vi "Get Service Description.vi"(0 "Room Service Base in":refnum<class "Room Service Base.lvclass">, 11 "error in (no error)":errorcluster) -> (4 "Room Service Base out":refnum<class "Room Service Base.lvclass">, 6 "Service Description":string, 15 "error out":errorcluster)   [LabVIEW 2023, in "Room Service Types.lvlib" / "Room Service Base.lvclass"]
uses:
  Room Service Base.lvclass
  Room Service Base.lvclass/Room Service Base.ctl
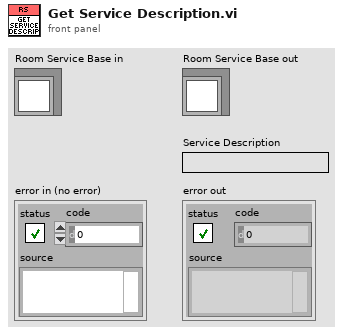
[diagram p1: front panel]
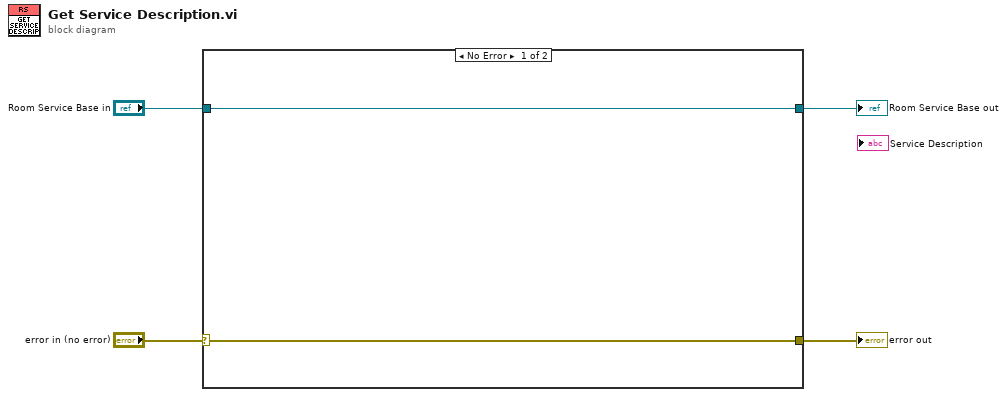
[diagram p0: block diagram]
diagram:
  n1 = case shown="No Error" "error in (no error)" {
    selector: "error in (no error)" -> [w5 w8]
    tunnel: [w5 w8] -> w3
    tunnel: [w6 w7] -> w1
    tunnel: "Room Service Base in" -> [w6 w7]
    frame No Error {
    }
    frame Error {
    }
  }
  "error out" <- w3
  "Room Service Base out" <- w1
